vi "View Subsystem IO Attributes Dialog.vi"(8 "error in (no error)":errorcluster) -> (0 "error out":errorcluster)   [LabVIEW 2024]
doc: "This VI is a user interface VI and is used to displays the subsystem configuration dialog and all the I/O attributes."
uses:
  Globals/Global - Server.vi
  <vilib>/Utility/file.llb/Read Delimited Spreadsheet (string).vi
panel:
  in  "Open":bool
  in  "Close":bool
  out "Subsystem I/O Attributes":i32(listbox)
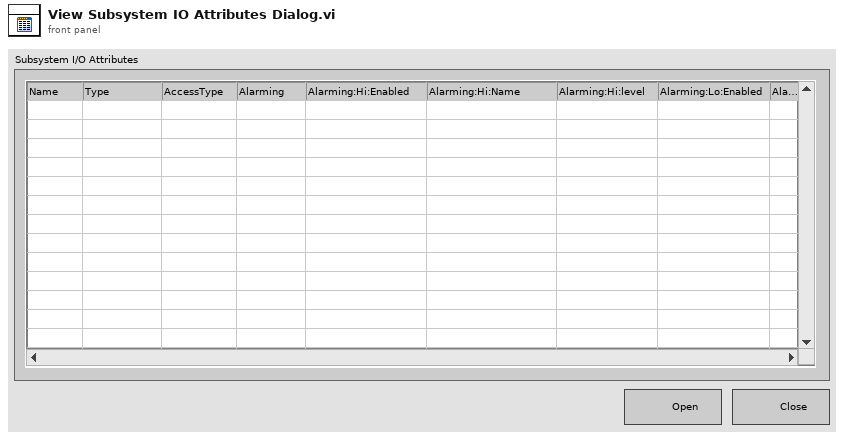
[diagram p1: front panel]
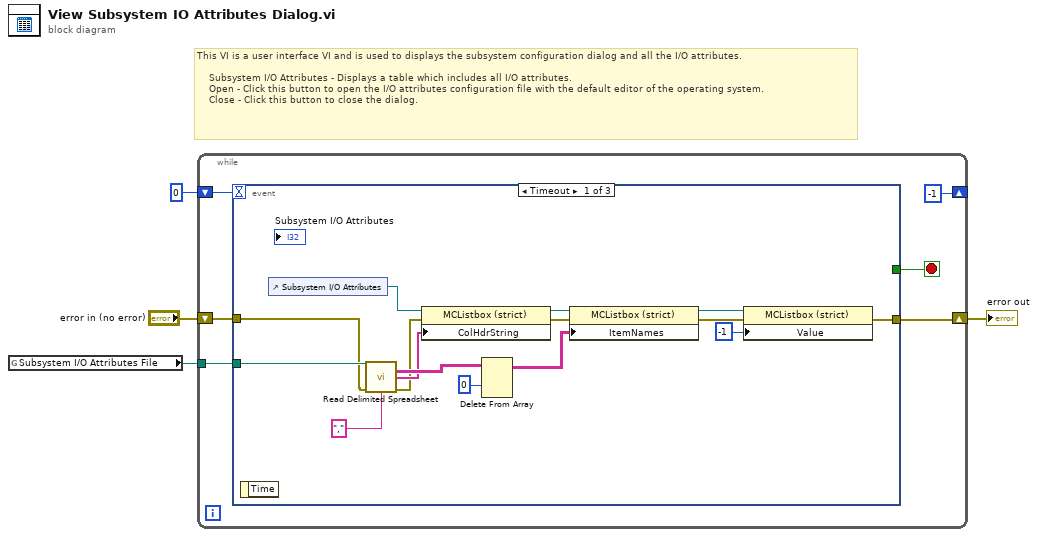
[diagram p0: block diagram]
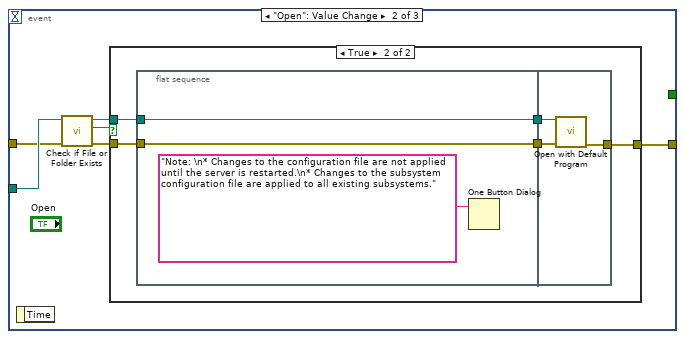
[diagram p2: hidden frame]
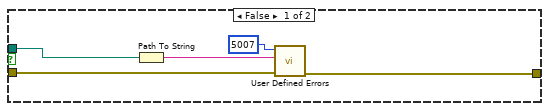
[diagram p3: hidden frame]
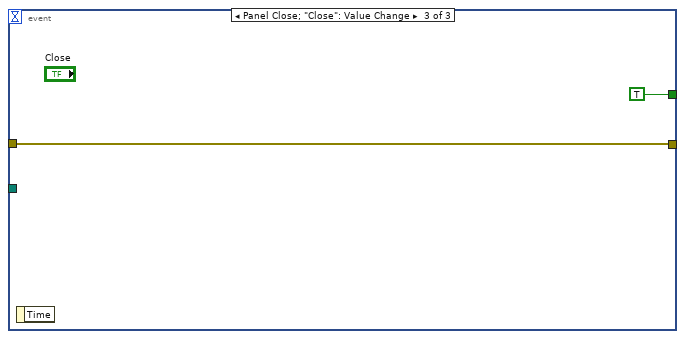
[diagram p4: hidden frame]
diagram:
  # "This VI is a user interface VI and is used to displays the subsystem configuration dialog and all the I/O attributes.\n\n    Subsystem I/O Attributes - Displays a table which includes all I/O attributes.\n    Open - Click this button to open the I/O attributes configuration file with the default editor of the operating system.  \n    Close - Click this button to close the dialog."
  n1 = global read "Global - Server.vi" "Subsystem I/O Attributes File"() -> (w3:path)
  n2 = while {
    shift-right: [-1] -> _
    shift-left: 0 -> [w9]
    tunnel: w3 -> [w8]
    shift-right: [w6] -> w1
    shift-left: "error in (no error)" -> [w7]
    stop <- w10 stop-if-true
    n3 = event shown="[0] Timeout" {
      selector: _ -> [_ _ _]
      dyn-events: _ -> [_ _ _]
      timeout: w9 -> [_ _ _]
      tunnel: [_ _ TRUE] -> w10
      tunnel: w8 -> [w18 w31 _]
      tunnel: w7 -> [w12 w26 w48]
      tunnel: [w14 w27 w48] -> w6
      event Timeout {
        n4 = event-data() -> ()  [unwired: 1 in, 1 out]
        n5 = control-ref of="Subsystem I/O Attributes"() -> (w24:refnum<vi>)
        n6 = call-poly <vilib>:"Read Delimited Spreadsheet.vi"("file path (dialog if empty)"=w18, "error in (no error)"=w12, "delimiter (\\t)"="," ("delimiter (\\t)")) -> ("all rows"=w21:string[][], "first row"=w13:string[], "error out"=w11:errorcluster)  [unwired: 7 in, 3 out]
        n7 = property on="Property Node" class="MCListbox (strict)"(reference=w24, error in=w11, "ColHdrString"=w13) -> (reference out=w25:refnum<vi>, error out=w23:errorcluster)
        n8 = Delete From Array(array=w21, index (row)=0) -> (array with subset deleted=w22:string[][])  [unwired: 2 in, 1 out]
        n9 = property on="Property Node" class="MCListbox (strict)"(reference=w25, error in=w23, "ItemNames"=w22) -> (reference out=w16:refnum<vi>, error out=w17:errorcluster)
        n10 = property on="Property Node" class="MCListbox (strict)"(reference=w16, error in=w17, "Value"=-1 ("index (row)")) -> (error out=w14:errorcluster)  [unwired: 1 out]
      }
      event "Open": Value Change {
        n11 = event-data() -> ()  [unwired: 1 in, 1 out]
        n12 = call <vilib>:"Check if File or Folder Exists.vi"("error in (no error)"=w26, "path"=w31) -> ("error out"=w28:errorcluster, "file or folder exists?"=w30:bool, "dup path"=w29:path)  [unwired: 7 in]
        n13 = case shown="True" w30 {
          tunnel: w29 -> [w36 w41]
          tunnel: w28 -> [w32 w40]
          tunnel: [w33 w39] -> w27
          frame False {
            n14 = Path To String(path=w36) -> (string=w35:string)
            n15 = call "User Defined Errors.vi"("error in (no error)"=w32, "Parameter 1"=w35, "Error Code (0)"=5007 ("error code (0)")) -> ("error out"=w33:errorcluster)  [unwired: 8 in]
          }
          frame True {
            n16 = flat-sequence {
              tunnel: w40 -> [w43]
              tunnel: w41 -> [w44]
              tunnel: [w44] -> w38
              tunnel: [w43] -> w37
              tunnel: [w45] -> w39
              tunnel: w38 -> [w47]
              tunnel: w37 -> [w46]
              frame #0 {
                n17 = One Button Dialog(message="Note: \n* Changes to the configuration file are not applied until the server is restarted.\n* Changes to the subsystem configuration file are applied to all existing subsystems.") -> ()  [unwired: 1 in, 1 out]
              }
              frame #1 {
                n18 = call "Open with Default Program.vi"("error in (no error)"=w46, "File Path"=w47) -> ("error out"=w45:errorcluster)  [unwired: 9 in]
              }
            }
          }
        }
      }
      event Panel Close; "Close": Value Change {
        n19 = event-data() -> ()  [unwired: 1 in, 1 out]
      }
    }
  }
  "error out" <- w1
